vi "User Interface.vi"(8 "error in (no error)":errorcluster, 11 "User Interface in":refnum<class "User Interface.lvclass">) -> (0 "error out":errorcluster, 3 "User Interface out":refnum<class "User Interface.lvclass">)   [LabVIEW 2017, in "DSF Core.lvlib" / "Settings Editor.lvclass"]
uses:
  Settings Editor.lvclass
  User Interface.lvclass
  C:/Git/DSF/Core/Classes/User Interface/User Interface.lvclass
  Settings Editor.lvclass/Settings Editor.ctl
  Plugin/Component Settings Editor.lvclass
  User Interface Handler/User Interface Handler.lvclass
panel:
  in  "Tab Control":enum32{"Core", "Components"}(tab)
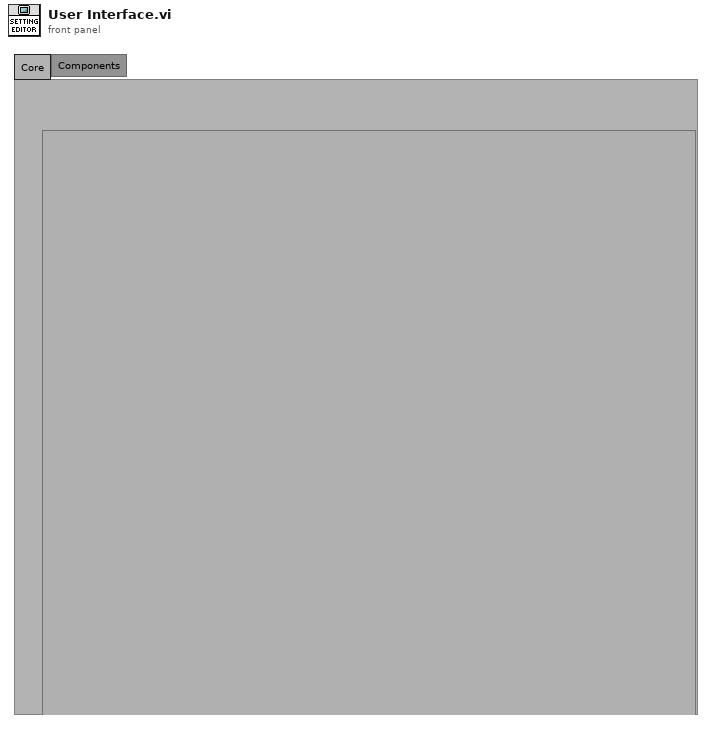
[diagram p1: front panel]
types:
  T1 = typedef "DSF Core.lvlib/User Interface Handler.lvclass/User Interface Ref.ctl" = refnum<vi>
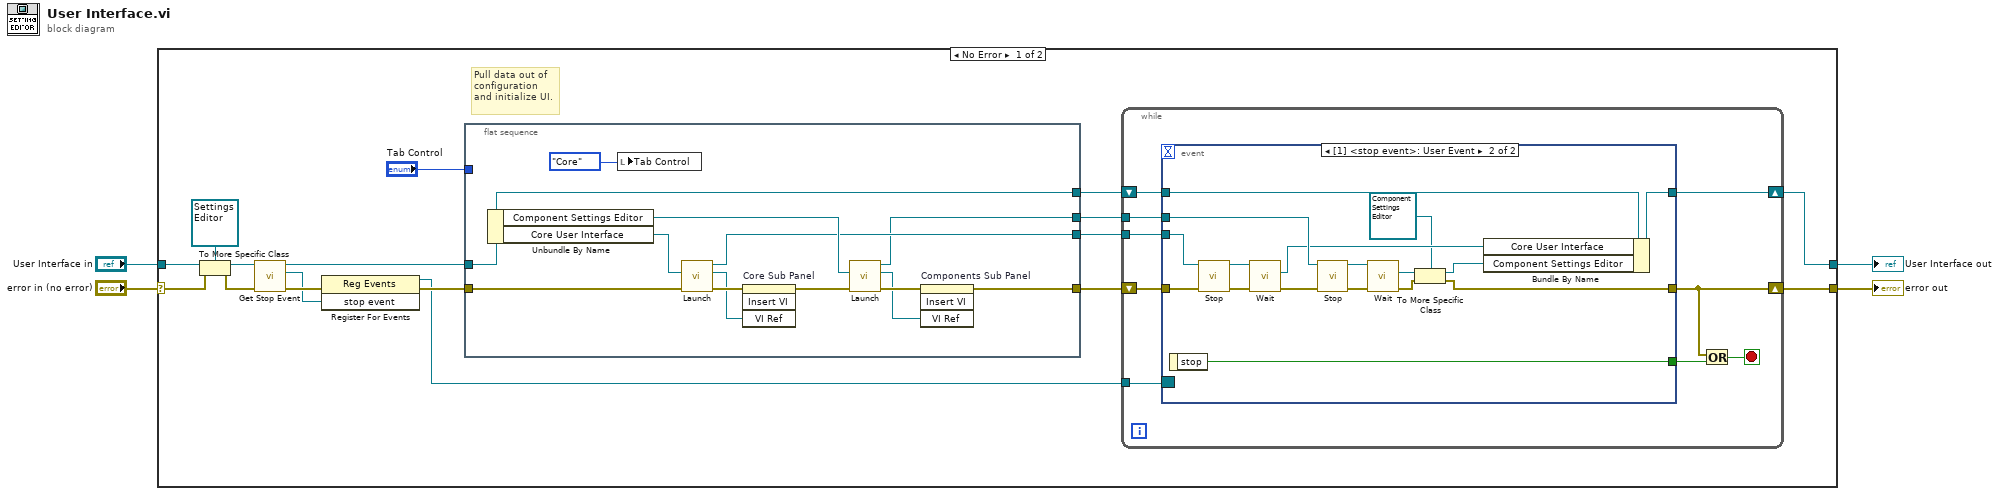
[diagram p0: block diagram]
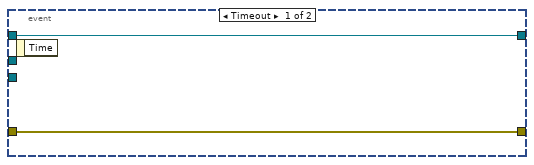
[diagram p2: hidden frame]
diagram:
  n1 = case shown="No Error" "error in (no error)" {
    selector: "error in (no error)" -> [w11 w64]
    tunnel: [w15 w64] -> w4
    tunnel: "User Interface in" -> [w13 w63]
    tunnel: [w14 w63] -> w1
    frame No Error {
      # "Pull data out of configuration and initialize UI."
      n2 = To More Specific Class(target class=refnum<class "Settings Editor.lvclass"> refnum ("DSF Core.lvlib:Settings Editor.lvclass"), reference=w13, error in=w11) -> (specific class reference=w12:refnum<class "Settings Editor.lvclass">, error out=w10:errorcluster)
      n3 = call "Get Stop Event.vi"("error in (no error)"=w10, "User Interface in"=w12) -> ("error out"=w20:errorcluster, "stop event"=w19:refnum<user-event>, "User Interface out"=w18:refnum<class "Settings Editor.lvclass">)  [unwired: 7 in]
      n4 = register-events(error in=w20, w19) -> (reference out=w16:refnum<event-registration>, error out=w17:errorcluster)  [unwired: 1 in]
      n5 = flat-sequence {
        tunnel: [w34] -> w21
        tunnel: w17 -> [w32]
        tunnel: w18 -> [w33]
        tunnel: [w33] -> w8
        tunnel: [w24] -> w7
        tunnel: [w23] -> w6
        tunnel: "Tab Control" -> [_]
        frame #0 {
          n6 = Unbundle By Name(w33) -> ("Component Settings Editor"=w27:refnum<class "Component Settings Editor.lvclass">, "Core User Interface"=w31:refnum<class "User Interface.lvclass">)
          n7 = local write "Tab Control"(enum32{"Core", "Components"}."Core" ("Tab Control")) -> ()
          n8 = call "Launch.vi"("error in (no error)"=w32, "User Interface"=w31) -> ("error out"=w30:errorcluster, "active vi"=w29:T1, "User Interface Handler out"=w24:refnum<class "User Interface Handler.lvclass">)  [unwired: 7 in]
          n9 = invoke on="Core Sub Panel" class="SubPnl" method="Insert VI"(error in=w30, "VI Ref"=w29) -> (error out=w28:errorcluster)  [unwired: 2 in, 3 out]
          n10 = call "Launch.vi"("error in (no error)"=w28, "User Interface"=w27) -> ("error out"=w26:errorcluster, "active vi"=w25:T1, "User Interface Handler out"=w23:refnum<class "User Interface Handler.lvclass">)  [unwired: 7 in]
          n11 = invoke on="Components Sub Panel" class="SubPnl" method="Insert VI"(error in=w26, "VI Ref"=w25) -> (error out=w34:errorcluster)  [unwired: 2 in, 3 out]
        }
      }
      n12 = while {
        tunnel: w16 -> [w43]
        shift-right: [w41] -> w15
        shift-left: w21 -> [w42]
        shift-right: [w37] -> w14
        shift-left: w8 -> [w38]
        tunnel: w7 -> [w36]
        tunnel: w6 -> [w35]
        stop <- w40 stop-if-true
        n13 = event shown="[1] <stop event>: User Event" {
          selector: w43 -> [_ _]
          dyn-events: _ -> [_ _]
          timeout: _ -> [_ _]
          tunnel: [_ w62] -> w39
          tunnel: w42 -> [w45 w61]
          tunnel: [w45 w46] -> w41
          tunnel: w38 -> [w44 w52]
          tunnel: [w44 w51] -> w37
          tunnel: w36 -> [_ w55]
          tunnel: w35 -> [_ w54]
          event Timeout {
            n14 = event-data() -> ()  [unwired: 1 in, 1 out]
          }
          event User Event {
            n15 = event-data() -> ("stop"=w62:bool)  [unwired: 1 in]
            n16 = call "Stop.vi"("error in (no error)"=w61, "User Interface Handler in"=w55) -> ("error out"=w60:errorcluster, "User Interface Handler out"=w59:refnum<class "User Interface Handler.lvclass">)  [unwired: 8 in]
            n17 = call "Wait.vi"("error in (no error)"=w60, "User Interface Handler in"=w59) -> ("error out"=w56:errorcluster, "User Interface"=w53:refnum<class "User Interface.lvclass">)  [unwired: 7 in, 1 out]
            n18 = call "Stop.vi"("error in (no error)"=w56, "User Interface Handler in"=w54) -> ("error out"=w58:errorcluster, "User Interface Handler out"=w57:refnum<class "User Interface Handler.lvclass">)  [unwired: 8 in]
            n19 = call "Wait.vi"("error in (no error)"=w58, "User Interface Handler in"=w57) -> ("error out"=w47:errorcluster, "User Interface"=w50:refnum<class "User Interface.lvclass">)  [unwired: 7 in, 1 out]
            n20 = To More Specific Class(target class=refnum<class "Component Settings Editor.lvclass"> refnum ("Component Settings Editor"), reference=w50, error in=w47) -> (specific class reference=w48:refnum<class "Component Settings Editor.lvclass">, error out=w46:errorcluster)
            n21 = Bundle By Name(cluster=w52, "Core User Interface"=w53, "Component Settings Editor"=w48) -> (w51:refnum<class "Settings Editor.lvclass">)
          }
        }
        n22 = Or(x=w41, y=w39) -> (x .or. y?=w40:bool)
      }
    }
    frame Error {
    }
  }
  "error out" <- w4
  "User Interface out" <- w1
